vi "Uninit.vi"(8 "error in":errorcluster, 11 "camera.nit in":refnum<class "camera.lvclass">) -> (0 "error out":errorcluster)   [LabVIEW 2020, in "camera.lvclass"]
uses:
  camera.lvclass
  camera.lvclass/camera.ctl
  lib/O-PL.dll
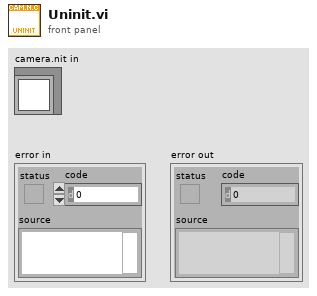
[diagram p1: front panel]
types:
  T1 = typedef "Semaphore RefNum" = refnum<k1>
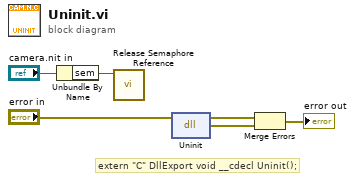
[diagram p0: block diagram]
diagram:
  # "extern \"C\" DllExport void __cdecl Uninit();"
  n1 = Unbundle By Name("camera.nit in") -> ("sem"=w3:T1)
  n2 = call <vilib>:"Release Semaphore Reference.vi"("semaphore"=w3) -> ()  [unwired: 9 in, 2 out]
  n3 = dll-call lib="C:/Users/pittsburger.SOLARIS/Desktop/v0.8/lib/O-PL.dll" fn="Uninit"() -> (error out=w5:errorcluster)  [unwired: 4 in, 1 out]
  n4 = Merge Errors("error in", w5) -> (→"error out":errorcluster)
